vi "DHE_DRV_get_imstatus.vi"(0 "fd":i32, 11 "error in (no error)":errorcluster) -> (1 "ptr to buffer":u64, 2 "image status":i16, 3 "exposure progress":i32, 4 "fd":i32, 6 "buff read":i32, 7 "fowlers_discarded":i32, 8 "frames read":i32, 9 "actual_buf_reads":i32, 10 "frame status":i32, 12 "coads_discarded":i32, 13 "coadds done":i32, 14 "images done":i32, 15 "error out":errorcluster)   [LabVIEW 2016]
doc: "This VI closes the I/O interface with the instrument."
uses:
  c/lib/libarcDHE.so
panel:
  in  "actual_bufers":i32
  in  "fowlers_disc":i32
  in  "coads_discar":i32
  in  "framestat":i32
  in  "coadds_done":i32
  in  "images_done":i32
  in  "imreads":i32
  in  "exp_prog":i32
  in  "imstat":i16
  in  "curr_ptr":u64
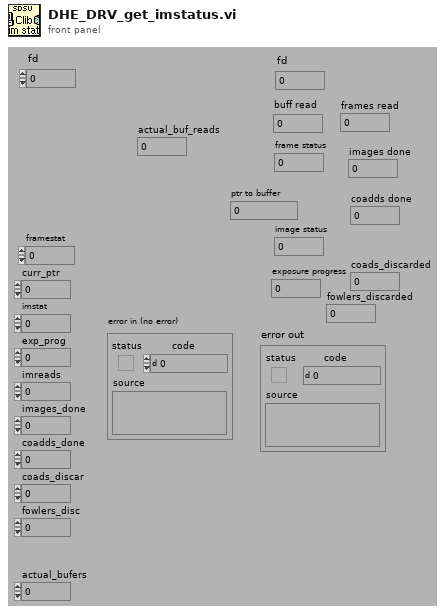
[diagram p1: front panel]
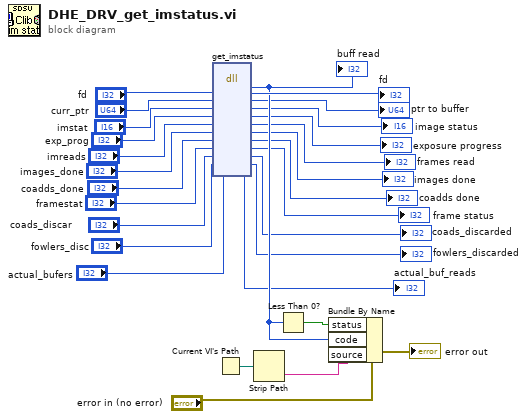
[diagram p0: block diagram]
diagram:
  n1 = dll-call lib="home/simager/panview/PAN/Modules/SDSU/private/c/lib/libarcDHE.so" fn="get_imstatus"("fd"="fd", "curr_ptr"="curr_ptr", "imstat"="imstat", "exp_prog"="exp_prog", "imreads"="imreads", "images_done"="images_done", "coadds_done"="coadds_done", "framestat"="framestat", "coads_discarded"="coads_discar", "fowler_discarded"="fowlers_disc", "actual_buf_reads"="actual_bufers") -> ("return type"=w21:i32, "fd"=→"fd":i32, "curr_ptr"=→"ptr to buffer":u64, "imstat"=→"image status":i16, "exp_prog"=→"exposure progress":i32, "imreads"=→"frames read":i32, "images_done"=→"images done":i32, "coadds_done"=→"coadds done":i32, "framestat"=→"frame status":i32, "coads_discarded"=→"coads_discarded":i32, "fowler_discarded"=→"fowlers_discarded":i32, "actual_buf_reads"=→"actual_buf_reads":i32)  [unwired: 3 in, 2 out]
  "buff read" <- w21
  n2 = Current VI's Path() -> (path=w26:path)
  n3 = Strip Path(path=w26) -> (name=w25:string)  [unwired: 1 out]
  n4 = Less Than 0?(x=w21) -> (x < 0?=w27:bool)
  n5 = Bundle By Name(cluster="error in (no error)", "status"=w27, "code"=w21, "source"=w25) -> (→"error out":errorcluster)
